vi "SimpleExample1_DS.vi"() -> ()   [LabVIEW 2011, in "Messenging.lvlib"]
uses:
  Messenging.lvlib
  Interprocess Messenger/Send/Send.lvclass
  Interprocess Messenger/Send/Send (no data).vi
  Interprocess Messenger/Send/Query (varients).vi
  Interprocess Messenger/DataSocketMessenger/DataSocketMessenger.lvclass
panel:
  out "Reply Label":string
  out "Time":timestamp
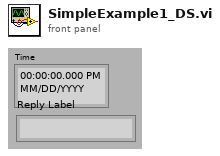
[diagram p1: front panel]
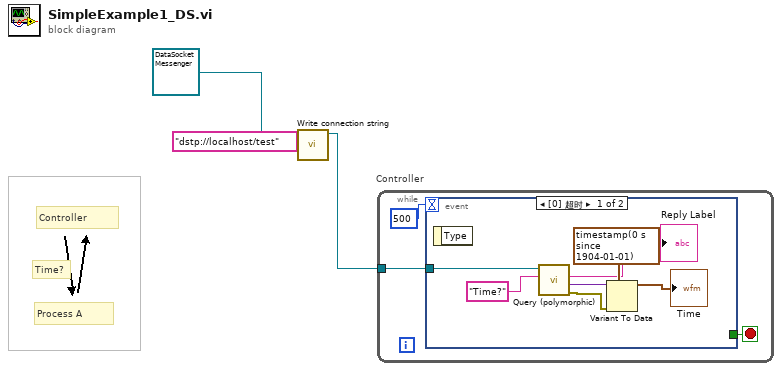
[diagram p0: block diagram]
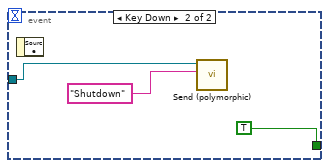
[diagram p2: hidden frame]
diagram:
  # "Time?"
  # "Process A"
  # "Controller"
  n1 = call-dynamic "Write connection string.vi"("connection string"="dstp://localhost/test", "DataSocketMessenger.lvclass in"=refnum<class "DataSocketMessenger.lvclass"> refnum ("Messenging.lvlib:DataSocketMessenger.lvclass")) -> ("DataSocketMessenger.lvclass out"=w1:refnum<class "DataSocketMessenger.lvclass">)  [unwired: 1 in, 8 out]
  n2 = while "Controller" {
    tunnel: w1 -> [w6]
    stop <- w5 stop-if-true
    n3 = event shown="[0] 超时" {
      selector: _ -> [_ _]
      dyn-events: _ -> [_ _]
      timeout: 500 -> [_ _]
      tunnel: w6 -> [w13 w15]
      tunnel: [_ TRUE] -> w5
      event Timeout {
        n4 = event-data() -> ()  [unwired: 2 out]
        n5 = call-poly "Query (polymorphic).vi"("Label"="Time?", "MSR Parent"=w13) -> ("error out"=w8:errorcluster, "Replay Varient"=w11:variant, "Reply Label"=→"Reply Label":string)  [unwired: 2 in, 5 out]
        n6 = Variant To Data(error in=w8, type=timestamp(0 s since 1904-01-01) ("current time"), Variant=w11) -> (data=→"Time":timestamp)  [unwired: 1 out]
      }
      event Key Down {
        n7 = event-data() -> ()  [unwired: 2 out]
        n8 = call-poly "Send (polymorphic).vi"("Label"="Shutdown", "MSR Parent in"=w15) -> ()  [unwired: 1 in, 9 out]
      }
    }
  }
